vi "I16-U16转换.vi"(1 "输入":i32[](array[numeric])) -> (0 "输出":i32[](array[numeric]))   [LabVIEW 2012]
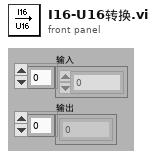
[diagram p1: front panel]
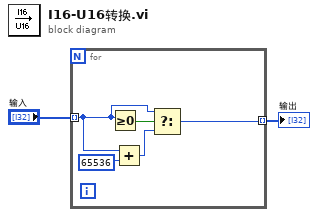
[diagram p0: block diagram]
diagram:
  n1 = for {
    tunnel: "输入" -> [w5] mode=indexing
    tunnel: [w6] -> w1 mode=indexing
    n2 = Greater Or Equal To 0?(x=w5) -> (x >= 0?=w7:bool)
    n3 = Add(x=w5, y=65536) -> (x+y=w3:i32)
    n4 = Select(t=w5, s=w7, f=w3) -> (s? t:f=w6:i32)
  }
  "输出" <- w1
